vi "Tabulator.vi"() -> ()   [LabVIEW 2024]
uses:
  Source/WebView_class/Editor Mode--enum.ctl
  Source/WebView.Tabulator_class/WebView.Tabulator.lvclass
  <vilib>/JDP Science/JSONtext/JSONtext.lvlib
  Source/WebView.JSONEditor_class/WebView.JSONEditor.lvclass
  <vilib>/sklein/WebView2/Libs/Microsoft.Web.WebView2.WinForms.dll
panel:
  in  "Mode":T1
  out "Error Out":errorcluster
  in  "System Load Button":bool
  in  "Stop":bool
  in  "Tab Control":enum32{"JSON", "JSON Schema"}(tab)
  in  "JSON (transparent)":string
  in  "JSON Schema":string
  in  "WebView2 Control in":refnum<k24>(container)
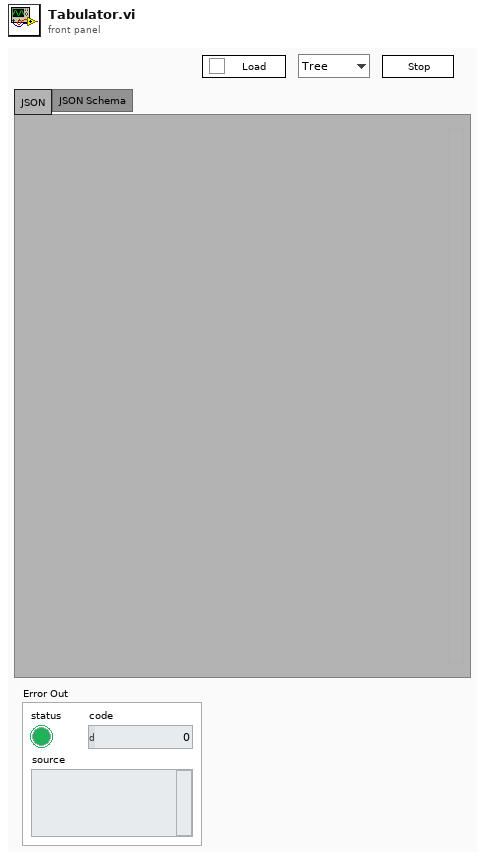
[diagram p1: front panel]
types:
  T1 = typedef "WebView.JSONEditor.lvclass/Editor Mode--enum.ctl" = enum16{"Tree", "View", "Form", "Code", "Text"}
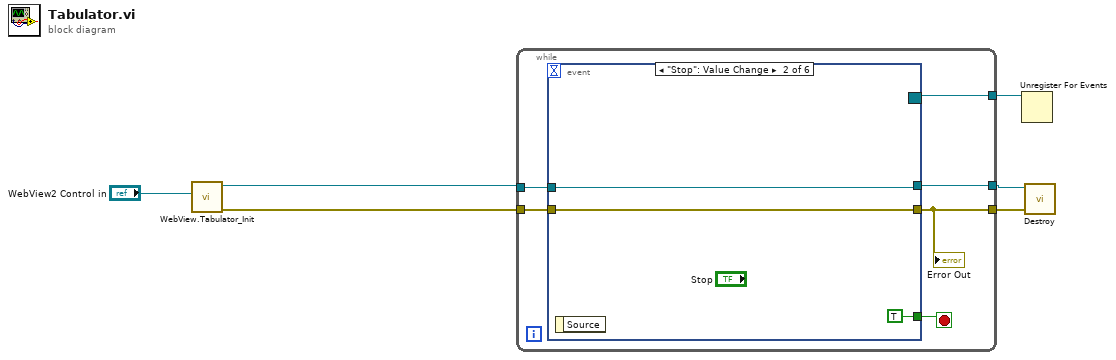
[diagram p0: block diagram]
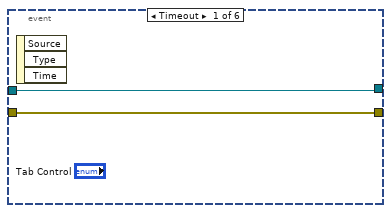
[diagram p2: hidden frame]
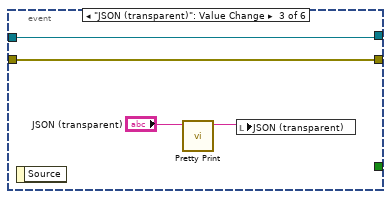
[diagram p3: hidden frame]
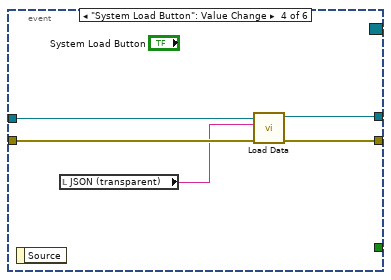
[diagram p4: hidden frame]
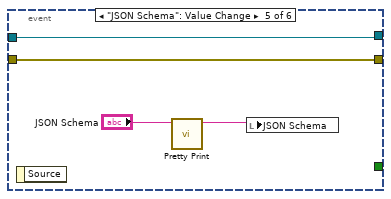
[diagram p5: hidden frame]
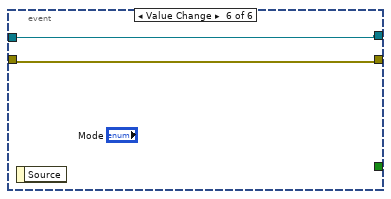
[diagram p6: hidden frame]
diagram:
  n1 = call "WebView.Tabulator_Init.vi"("WebView2 Control in"="WebView2 Control in") -> ("Error Out"=w4:errorcluster, "object out"=w5:refnum<class "WebView.Tabulator.lvclass">)  [unwired: 9 in]
  n2 = while {
    tunnel: w5 -> [w12]
    tunnel: w4 -> [w11]
    tunnel: [w8] -> w1
    tunnel: [w10] -> w2
    tunnel: [w7] -> w6
    stop <- w9 stop-if-true
    n3 = event shown="[1] \"Stop\": Value Change" {
      selector: _ -> [_ _ _ _ _ _]
      dyn-events: [_ _ _ _ _ _] -> w7
      timeout: _ -> [_ _ _ _ _ _]
      tunnel: w12 -> [w14 w15 w19 w24 w28 w31]
      tunnel: w11 -> [w13 w16 w18 w26 w27 w32]
      tunnel: [w13 w16 w18 w25 w27 w32] -> w8
      tunnel: [w14 w15 w19 w23 w28 w31] -> w10
      tunnel: [_ TRUE _ _ _ _] -> w9
      event Timeout {
        n4 = event-data() -> ()  [unwired: 1 in, 3 out]
      }
      event "Stop": Value Change {
        n5 = event-data() -> ()  [unwired: 1 in, 1 out]
      }
      event "JSON (transparent)": Value Change {
        n6 = event-data() -> ()  [unwired: 1 in, 1 out]
        n7 = call <vilib>:"Pretty Print.vi"("JSON"="JSON (transparent)") -> ("<JSON>"=w20:string)  [unwired: 8 in, 2 out]
        n8 = local write "JSON (transparent)"(w20) -> ()
      }
      event "System Load Button": Value Change {
        n9 = event-data() -> ()  [unwired: 1 in, 1 out]
        n10 = local read "JSON (transparent)"() -> (w22:string)
        n11 = call-dynamic "Load Data.vi"("Error In"=w26, "<JSON> in"=w22, "object in"=w24) -> ("Error Out"=w25:errorcluster, "object out"=w23:refnum<class "WebView.Tabulator.lvclass">)  [unwired: 7 in]
      }
      event "JSON Schema": Value Change {
        n12 = event-data() -> ()  [unwired: 1 in, 1 out]
        n13 = call <vilib>:"Pretty Print.vi"("JSON"="JSON Schema") -> ("<JSON>"=w29:string)  [unwired: 8 in, 2 out]
        n14 = local write "JSON Schema"(w29) -> ()
      }
      event Value Change {
        n15 = event-data() -> ()  [unwired: 1 in, 1 out]
      }
    }
    "Error Out" <- w8
  }
  n16 = Unregister For Events(event registration refnum=w6) -> ()  [unwired: 1 in, 1 out]
  n17 = call-dynamic "Destroy.vi"("Error In"=w1, "Object in"=w2) -> ()  [unwired: 9 in, 1 out]
